vi "haomain.vi"() -> ()   [LabVIEW 2018]
uses:
  <vilib>/Platform/TimedLoop/XDataNode/timing_clust.ctl
  <vilib>/Platform/TimedLoop/XDataNode/nitl_modes.ctl
  <vilib>/Platform/TimedLoop/XDataNode/wakeup.ctl
  <vilib>/FPGAPlugInAG/myRIO-1900/niLvFpga_Open_myRIO-1900.vi
  <vilib>/rvi/interface/common/dynamic/niFpgaDynamicAddResources.vi
  <vilib>/Utility/error.llb/Error Cluster From Error Code.vi
  <vilib>/rvi/errors/niLvFpgaAdjustHostInterfaceError.vi
  <vilib>/rvi/interface/nirviOpenFPGA/nirviOpenFPGA.xnode
  FPGA Bitfiles/Dentalrobot_FPGATarget_DIOtest_chEYOcGDYLI.lvbitx
  FPGA/DIO test.vi
  <vilib>/rvi/interface/nirviReadWriteControl/nirviReadWriteControl.xnode
  <vilib>/Platform/TimedLoop/XDataNode/XDataNode.xnode
  <vilib>/Platform/TimedLoop/XDataNode/XDNodeRunTimeDep.lvlib
  <vilib>/rvi/interface/Simulation/niFpgaSimulationCallBeginRW.vi
  NiFpgaLv.dll
panel:
  in  "DC":fxp<+,32,0>
  in  "stop":bool
  out "C":bool
  in  "B":bool
  in  "A":bool
  out "finish delay":dbl
  out "Signal":bool[](array[boolean])
  in  "Steps/round":u32=200 step=2
  in  "Mode":string(combo)="4"
  in  "RPM":string(combo)="150"
  in  "move  (step)":i32 step=100
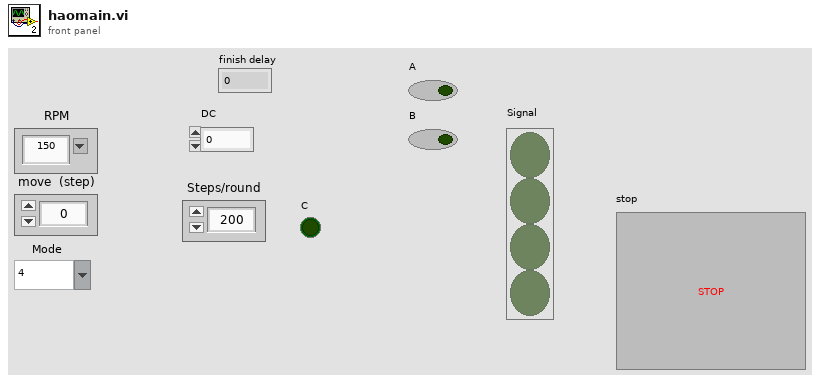
[diagram p1: front panel]
types:
  T1 = typedef "XDNodeRunTimeDep.lvlib/timing_clust.ctl" = cluster{"Expected End [f-1]":u64, "Actual End [f-1]":u64, "Finished Late? [f-1]":bool, "Expected End [i-1]":u64, "Actual End [i-1]":u64, "Finished Late? [i-1]":bool, "Expected Start [i]":u64, "Actual Start [i]":u64, "Expected Start [f]":u64, "Actual Start [f]":u64, "Source Name":string, "Structure Name":string, "Period":i64, "Deadline":i64, "Offset":i64, "Start":i64, "Priority":i32, "Timeout":i32, "Mode":T2, "Wakeup Reason":T3, "Error":errorcluster, "Source Type":string, "Secondary Source Type":string, "Global End Time":u64, "Global Start Time":u64, "Frame Duration":u64, "Iteration Duration":u64, "Assigned CPU":i32, "I/O Scan Engine Mode":u32}
  T2 = typedef "XDNodeRunTimeDep.lvlib/nitl_modes.ctl" = enum32{"No Change", "Process missed periods, maintain original phase", "Discard missed periods, maintain original phase", "Process missed periods, ignore original phase", "Discard missed periods, ignore original phase"}
  T3 = typedef "XDNodeRunTimeDep.lvlib/wakeup.ctl" = enum32{"Normal", "Aborted", "Asynchronous wakeup", "Timing source error", "Timed loop error", "Timeout"}
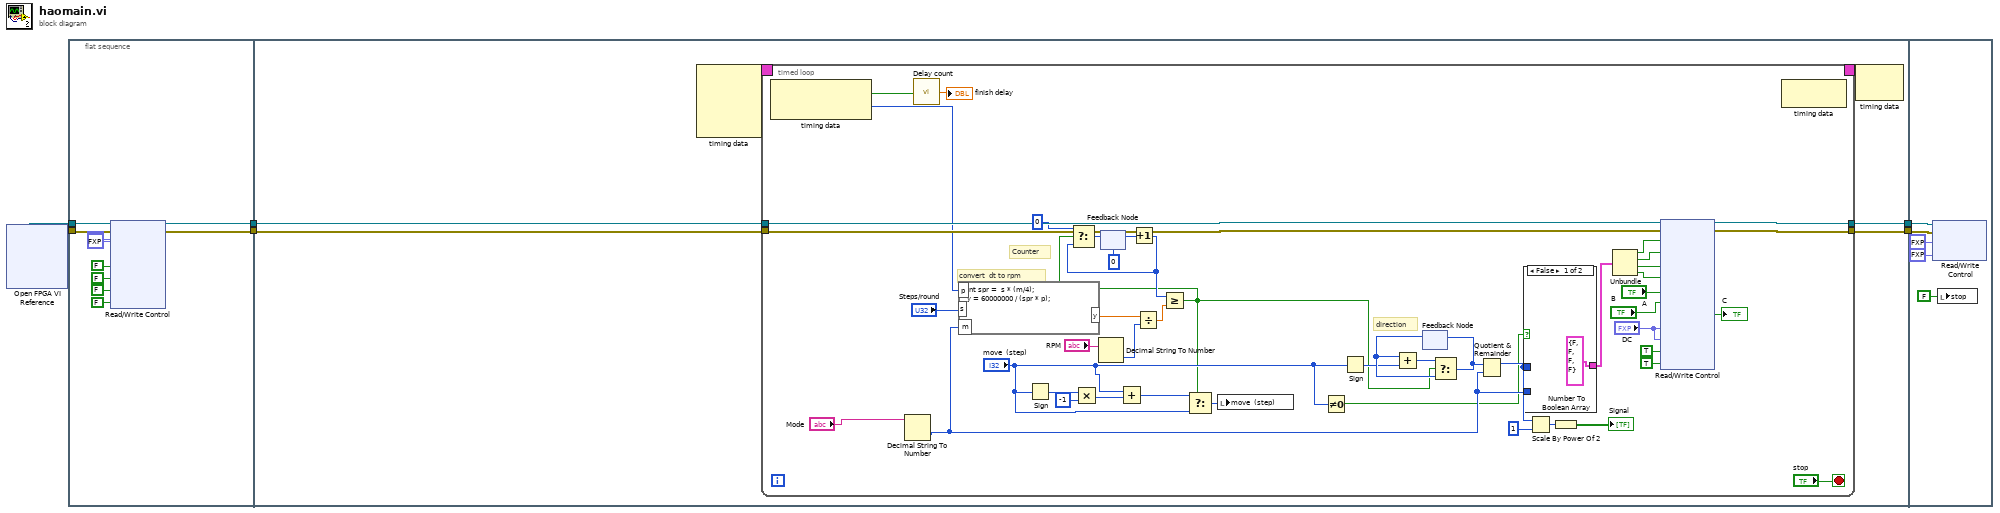
[diagram p0: block diagram]
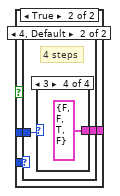
[diagram p2: hidden frame]
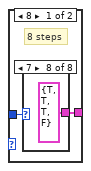
[diagram p3: hidden frame]
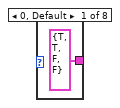
[diagram p4: hidden frame]
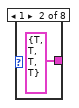
[diagram p5: hidden frame]
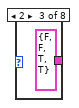
[diagram p6: hidden frame]
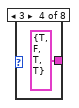
[diagram p7: hidden frame]
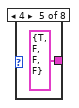
[diagram p8: hidden frame]
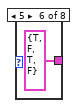
[diagram p9: hidden frame]
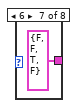
[diagram p10: hidden frame]
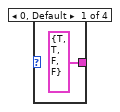
[diagram p11: hidden frame]
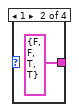
[diagram p12: hidden frame]
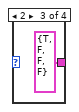
[diagram p13: hidden frame]
diagram:
  n1 = xnode "Open FPGA VI Reference"() -> ("FPGA VI Reference Out"=w6:refnum<k20>, "error out"=w5:errorcluster)  [unwired: 2 in]
  n2 = flat-sequence {
    tunnel: w6 -> [w16]
    tunnel: w5 -> [w15]
    tunnel: [w14] -> w4
    tunnel: [w13] -> w3
    tunnel: w4 -> [w20]
    tunnel: w3 -> [w19]
    tunnel: [w18] -> w2
    tunnel: [w17] -> w1
    tunnel: w2 -> [w100]
    tunnel: w1 -> [w99]
    frame #0 {
      n3 = xnode "Read/Write Control"("FPGA VI Reference In"=w16, "error in"=w15, "CH1 DC"=fxp<+,32,0> 0.0, "CH2 DC"=fxp<+,32,0> 0.0, "STBY2"=FALSE, "ENA2"=FALSE, "DIR2"=FALSE, "stop"=FALSE) -> ("FPGA VI Reference Out"=w14:refnum<k20>, "error out"=w13:errorcluster)
    }
    frame #1 {
      n4 = node-c288() -> (w22:T1)  [unwired: 4 in]
      n5 = timed-loop {
        timing: w22 -> [_]
        timing-out: [_] -> w21
        tunnel: w20 -> [w69]
        tunnel: w19 -> [w68]
        tunnel: [w67] -> w18
        tunnel: [w66] -> w17
        stop <- "stop" stop-if-true
        # "direction"
        # "Counter"
        # "convert  dt to rpm"
        n6 = node-c288() -> (w42:bool, w43:i64)  [unwired: 1 in]
        n7 = Decimal String To Number(string="Mode") -> (number=w32:i32)  [unwired: 2 in, 1 out]
        n8 = call "Delay count.vi"("Finished Late? [i-1]"=w42) -> ("Count"=→"finish delay":dbl)
        n9 = formula code="int spr =  s * (m/4); \ny = 60000000 / (spr * p);"("s"="Steps/round", "p"=w43, "m"=w32) -> ("y"=w54:dbl)
        n10 = Sign(1:"move  (step)") -> (0:w56:i32)
        n11 = Multiply(x=w56, y=-1) -> (x*y=w58:i32)
        n12 = Decimal String To Number(string="RPM") -> (number=w53:i32)  [unwired: 2 in, 1 out]
        n13 = feedback #1(0) -> (w46:i32)
        n14 = Add(x="move  (step)", y=w58) -> (x+y=w57:i32)
        n15 = Increment(x=w46) -> (x+1=w47:i32)
        n16 = Divide(x=w54, y=w53) -> (x/y=w52:dbl)
        n17 = Greater Or Equal?(x=w47, y=w52) -> (x >= y?=w23:bool)
        n18 = Select(t=0, s=w23, f=w47) -> (s? t:f=w45:i32)
        n19 = feedback-in #1(w45) -> ()
        n20 = Select(t=w57, s=w23, f="move  (step)") -> (s? t:f=w55:i32)
        n21 = local write "move  (step)"(w55) -> ()
        n22 = Not Equal To 0?(x="move  (step)") -> (x != 0?=w24:bool)
        n23 = Sign(1:"move  (step)") -> (0:w61:i32)
        n24 = feedback #2() -> (w62:i32)  [unwired: 1 in]
        n25 = Add(x=w62, y=w61) -> (x+y=w60:i32)
        n26 = Select(t=w60, s=w23, f=w62) -> (s? t:f=w63:i32)
        n27 = feedback-in #2(w63) -> ()
        n28 = Quotient & Remainder(x=w63, y=w32) -> (x-y*floor(x/y)=w31:i32)  [unwired: 1 out]
        n29 = case shown="False" w24 {
          tunnel: [cluster{bool, bool, bool, bool} {FALSE, FALSE, FALSE, FALSE} w73] -> w64
          tunnel: w32 -> [_ w72]
          tunnel: w31 -> [_ w71]
          frame False {
          }
          frame True {
            n30 = case shown="4, Default" w72 {
              tunnel: [w75 w85] -> w73
              tunnel: w71 -> [w74 w84]
              frame 8 {
                # "8 steps"
                n31 = case shown="7" w74 {
                  tunnel: [cluster{bool, bool, bool, bool} {TRUE, TRUE, FALSE, FALSE} cluster{bool, bool, bool, bool} {TRUE, TRUE, TRUE, TRUE} cluster{bool, bool, bool, bool} {FALSE, FALSE, TRUE, TRUE} cluster{bool, bool, bool, bool} {TRUE, FALSE, TRUE, TRUE} cluster{bool, bool, bool, bool} {TRUE, FALSE, FALSE, FALSE} cluster{bool, bool, bool, bool} {TRUE, FALSE, TRUE, FALSE} cluster{bool, bool, bool, bool} {FALSE, FALSE, TRUE, FALSE} cluster{bool, bool, bool, bool} {TRUE, TRUE, TRUE, FALSE}] -> w75
                  frame 0, Default {
                  }
                  frame 1 {
                  }
                  frame 2 {
                  }
                  frame 3 {
                  }
                  frame 4 {
                  }
                  frame 5 {
                  }
                  frame 6 {
                  }
                  frame 7 {
                  }
                }
              }
              frame 4, Default {
                # "4 steps"
                n32 = case shown="3" w84 {
                  tunnel: [cluster{bool, bool, bool, bool} {TRUE, TRUE, FALSE, FALSE} cluster{bool, bool, bool, bool} {FALSE, FALSE, TRUE, TRUE} cluster{bool, bool, bool, bool} {TRUE, FALSE, FALSE, FALSE} cluster{bool, bool, bool, bool} {FALSE, FALSE, TRUE, FALSE}] -> w85
                  frame 0, Default {
                  }
                  frame 1 {
                  }
                  frame 2 {
                  }
                  frame 3 {
                  }
                }
              }
            }
          }
        }
        n33 = Scale By Power Of 2(n=w31, x=u32 1) -> (x*2^n=w51:u32)
        n34 = Number To Boolean Array(number=w51) -> (Boolean array=→"Signal":bool[])
        n35 = Unbundle(w64) -> (w40:bool, w39:bool, w38:bool, w37:bool)
        n36 = xnode "Read/Write Control"("FPGA VI Reference In"=w69, "error in"=w68, "ENA1"=w40, "DIR1"=w39, "ENA2"=w38, "DIR2"=w37, "A"="A", "B"="B", "CH1 DC"="DC", "CH2 DC"="DC", "STBY2"=TRUE, "STBY1"=TRUE) -> ("FPGA VI Reference Out"=w67:refnum<k20>, "error out"=w66:errorcluster, "C"=→"C":bool)
        n37 = node-c288() -> ()  [unwired: 1 in, 1 out]
      }
      n38 = node-c288(w21) -> ()  [unwired: 1 out]
    }
    frame #2 {
      n39 = xnode "Read/Write Control"("FPGA VI Reference In"=w100, "error in"=w99, "CH1 DC"=fxp<+,32,0> 0.0, "CH2 DC"=fxp<+,32,0> 0.0) -> ()  [unwired: 2 out]
      n40 = local write "stop"(FALSE ("stop")) -> ()
    }
  }
